vi "Select element.vi"(9 "index":i32, 10 "unsigned byte array":u8[](array[numeric])) -> (2 "Numeric":u32)   [LabVIEW 2010]
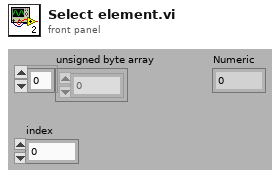
[diagram p1: front panel]
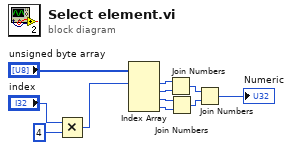
[diagram p0: block diagram]
diagram:
  n1 = Multiply(x="index", y=4) -> (x*y=w1:i32)
  n2 = Index Array(array="unsigned byte array", index #1=w1) -> (element #1=w5:u8, element #2=w6:u8, element #3=w7:u8, element #4=w8:u8)  [unwired: 3 in]
  n3 = Join Numbers(hi=w5, lo=w6) -> ((hi.lo)=w10:u16)
  n4 = Join Numbers(hi=w7, lo=w8) -> ((hi.lo)=w9:u16)
  n5 = Join Numbers(hi=w10, lo=w9) -> ((hi.lo)=→"Numeric":u32)
